vi "PLC Sim Launcher.vi"() -> ()   [LabVIEW 2019]
uses:
  PLC Sim Controller/PLC Sim Controller/PLC Sim Controller Actor.lvclass
  C:/Program Files (x86)/National Instruments/LabVIEW 2019/vi.lib/ActorFramework/Actor/Actor.lvclass
  f3c1f790-3e5d-4544-8d8b-87c596bc95fa.vi
  <vilib>/ActorFramework/Actor/Actor.lvclass
panel:
  out "Waiting Lights":T1
  # "PLC Simulated Server"
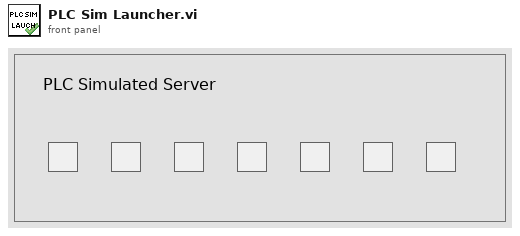
[diagram p1: front panel]
types:
  T1 = cluster{"Wait 1":bool, "Wait 2":bool, "Wait 3":bool, "Wait 4":bool, "Wait 5":bool, "Wait 6":bool, "Wait 7":bool}
  T2 = cluster{"[0]":bool, "[1]":bool, "[2]":bool, "[3]":bool, "[4]":bool, "[5]":bool, "[6]":bool}
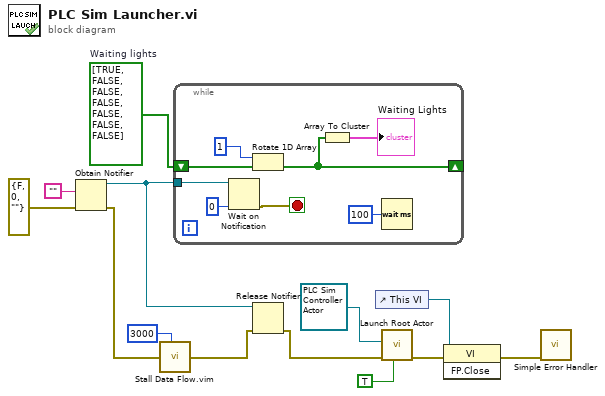
[diagram p0: block diagram]
diagram:
  w10 = bool[] [TRUE, FALSE, FALSE, FALSE, FALSE, FALSE, FALSE]  # Waiting lights
  n1 = Obtain Notifier(notification data type="", error in (no error)=errorcluster {"status"=FALSE, "code"=0, "source"=""}) -> (notifier out=w7:refnum<notifier>, error out=w6:errorcluster)  [unwired: 2 in, 1 out]
  n2 = call "Stall Data Flow.vim"("value in"=w6, "milliseconds to wait"=u32 3000) -> ("value out"=w11:errorcluster)  [unwired: 1 out]
  n3 = while {
    shift-right: [w15] -> _
    shift-left: w10 -> [w17]
    tunnel: w7 -> [w19]
    stop <- w21 stop-if-true
    n4 = Wait on Notification(notifier=w19, timeout in ms (-1)=0) -> (error out=w21:errorcluster)  [unwired: 2 in, 3 out]
    n5 = Rotate 1D Array(1:w17, 2:1 ("n")) -> (0:w15:bool[])
    n6 = Array To Cluster(array=w15) -> (cluster=→"Waiting Lights":T2)
    n7 = Wait (ms)(milliseconds to wait=u32 100) -> ()  [unwired: 1 out]
  }
  n8 = Release Notifier(notifier=w7, error in (no error)=w11) -> (error out=w5:errorcluster)  [unwired: 1 in, 2 out]
  n9 = control-ref of="This VI"() -> (w1:refnum<vi>)
  n10 = call <vilib>:"Launch Root Actor.vi"("Open Actor Core front panel? (F)"=TRUE, "error in (no error)"=w5, "Actor"=refnum<class "PLC Sim Controller Actor.lvclass"> refnum ("PLC Sim Controller Actor.lvlib:PLC Sim Controller Actor.lvclass")) -> ("error out"=w4:errorcluster)  [unwired: 7 in, 1 out]
  n11 = invoke class="VI" method="FP.Close"(reference=w1, error in=w4) -> (error out=w2:errorcluster)  [unwired: 1 in, 2 out]
  n12 = call <vilib>:"Simple Error Handler.vi"("error in (no error)"=w2) -> ()  [unwired: 4 in, 5 out]
